vi "获取最新一笔数据.vi"(7 "数据库类型":T1, 8 "错误输入（无错误）":errorcluster, 9 "Password":string, 10 "ping":bool, 11 "table":string) -> (0 "错误输出":errorcluster, 2 "检测值":cluster{"时间":timestamp, "检测值":dbl}, 3 "data":dbl)   [LabVIEW 2016]
uses:
  <vilib>/LabVIEW Open Source Project/OpenSerializer.Base64/Base64_CharSet.vi
  <vilib>/addons/database/Connection.llb/DB Tools Open Connec (String).vi
  <vilib>/addons/database/Connection.llb/Conn Execute.vi
  <vilib>/addons/database/Recordset.llb/Rec Fetch Recordset Data (R).vi
  <vilib>/addons/database/Recordset.llb/Rec Destroy - Connection.vi
  <userlib>/_LVST/sqlite_api/Core/Query/SQLite_Query-Standard.vi
  <vilib>/addons/database/_DB Variant To Data/Database Variant To Data.xnode
  <vilib>/addons/database/NI_Database_API.lvlib
  SQLite/SQLite Lib.lvlib
  Access/Access Lib.lvlib
  <vilib>/LabVIEW Open Source Project/OpenSerializer.Base64/Serializer.Base64.lvclass
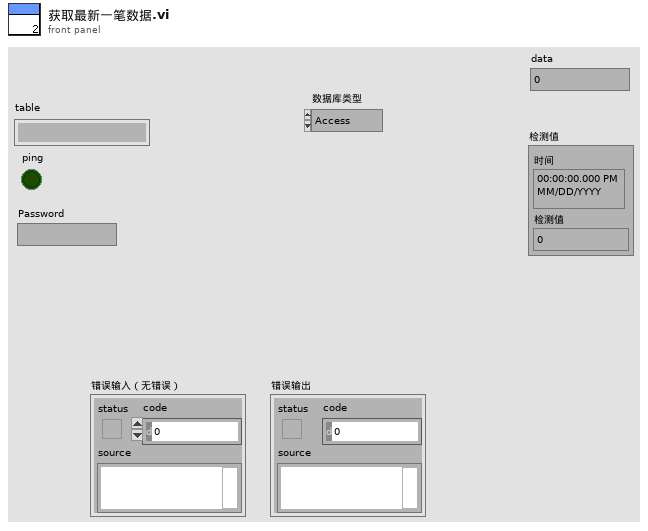
[diagram p1: front panel]
types:
  T1 = typedef "数据库类型.ctl" = enum16{"Access", "SQLite"}
  T2 = typedef "NI_Database_API.lvlib/Conn ObjectReference.ctl" = refnum<k1>
  T3 = typedef "NI_Database_API.lvlib/Rec ObjectReference.ctl" = refnum<k1>
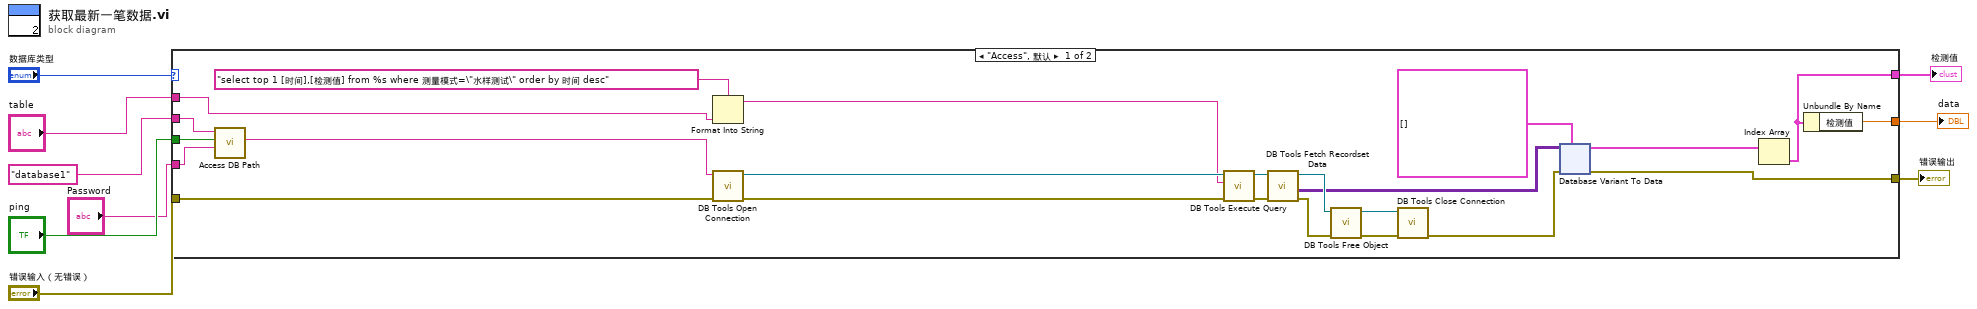
[diagram p0: block diagram]
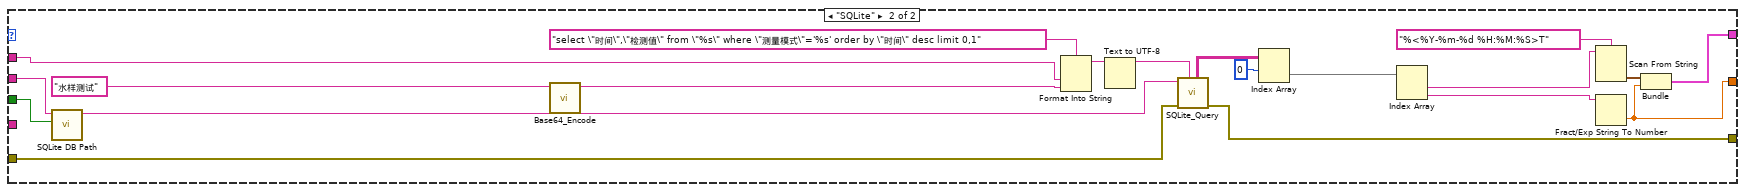
[diagram p2: hidden frame]
diagram:
  n1 = case shown="\"Access\", 默认" "数据库类型" {
    tunnel: "table" -> [w32 w134]
    tunnel: [w13 w128] -> w8
    tunnel: "错误输入（无错误）" -> [w21 w131]
    tunnel: [w19 w132] -> w6
    tunnel: "database1" ("database") -> [w18 w136]
    tunnel: [w14 w126] -> w3
    tunnel: "ping" -> [w12 w121]
    tunnel: "Password" -> [w10 _]
    frame "Access", Default {
      n2 = call "Access DB Path.vi"("Password"=w10, "ping"=w12, "database"=w18) -> ("Connection information"=w11:string)  [unwired: 7 in, 1 out]
      n3 = Format Into String(format string="select top 1 [时间],[检测值] from %s where 测量模式=\"水样测试\" order by 时间 desc" ("格式字符串"), w32) -> (resulting string=w22:string)  [unwired: 2 in, 1 out]
      n4 = call-poly <vilib>:"DB Tools Open Connection.vi"("error in (no error)"=w21, "connection information"=w11) -> ("error out"=w26:errorcluster, "connection reference"=w27:T2)  [unwired: 6 in]
      n5 = call-poly <vilib>:"DB Tools Execute Query.vi"("error in (no error)"=w26, "SQL query"=w22, "connection reference"=w27) -> ("error out"=w25:errorcluster, "recordset reference"=w30:T3)  [unwired: 5 in]
      n6 = call-poly <vilib>:"DB Tools Fetch Recordset Data.vi"("error in (no error)"=w25, "recordset reference"=w30) -> ("error out"=w28:errorcluster, "recordset data"=w16:variant[][], "recordset reference out"=w29:T3)  [unwired: 3 in]
      n7 = call-poly <vilib>:"DB Tools Free Object.vi"("error in (no error)"=w28, "recordset reference"=w29) -> ("error out"=w23:errorcluster, "connection reference"=w24:T2)  [unwired: 8 in]
      n8 = call <vilib>:"DB Tools Close Connection.vi"("error in (no error)"=w23, "connection reference"=w24) -> ("error out"=w20:errorcluster)  [unwired: 5 in]
      n9 = xnode "Database Variant To Data"("database variant"=w16, "error in (no error)"=w20, "type"=cluster{"时间":timestamp, "检测值":dbl}[] []) -> ("data"=w15:cluster{"时间":timestamp, "检测值":dbl}[], "error out"=w19:errorcluster)
      n10 = Index Array(array=w15) -> (element=w14:cluster{"时间":timestamp, "检测值":dbl})  [unwired: 1 in]
      n11 = Unbundle By Name(w14) -> ("检测值"=w13:dbl)
    }
    frame "SQLite" {
      n12 = call "SQLite DB Path.vi"("ping"=w121, "database"=w136) -> ("Path out"=w137:string)  [unwired: 9 in]
      n13 = call <vilib>:"Base64_Encode.vi"("String"="水样测试") -> ("Encoded String"=w119:string)  [unwired: 9 in, 1 out]
      n14 = Format Into String(format string="select \"时间\",\"检测值\" from \"%s\" where \"测量模式\"='%s' order by \"时间\" desc limit 0,1" ("格式字符串"), w134, w119) -> (resulting string=w124:string)  [unwired: 2 in, 1 out]
      n15 = Text to UTF-8(11:w124) -> (3:w123:string)  [unwired: 2 in, 1 out]
      n16 = call-poly <userlib>:"SQLite_Query.vi"("SQL Query"=w123, "error in (no error)"=w131, "DB Path"=w137) -> ("error out"=w132:errorcluster, "Results"=w122:string[][])  [unwired: 3 in, 2 out]
      n17 = Index Array(array=w122, index (row)=0 ("索引 (行)")) -> (element=w118:string[])  [unwired: 1 in]
      n18 = Index Array(array=w118) -> (element #1=w125:string, element #2=w130:string)  [unwired: 2 in]
      n19 = Scan From String(format string="%<%Y-%m-%d %H:%M:%S>T" ("格式字符串"), input string=w125) -> (output 1=w127:timestamp)  [unwired: 3 in, 3 out]
      n20 = Fract/Exp String To Number(string=w130) -> (number=w128:dbl)  [unwired: 3 in, 1 out]
      n21 = Bundle(w127, w128) -> (w126:cluster{timestamp, dbl})  [unwired: 1 in]
    }
  }
  "错误输出" <- w6
  "data" <- w8
  "检测值" <- w3
